vi "ReadTrajectory_JSON_File_WriteFGV_Example.vi"() -> ()   [LabVIEW 2019]
panel:
  out "error out":errorcluster
  # "Read Trajectory JSON File and Write to Functional Global Variable"
  # "See block diagram"
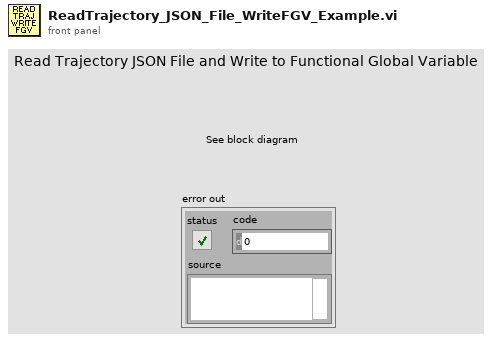
[diagram p1: front panel]
types:
  T1 = enum16{"Sample Fwd", "Sample Rev", "Read Traj", "Write Traj"}
  T2 = typedef "Trajectory_Library.lvlib/TRAJECTORY.ctl" = cluster{"TotalTImeSecs":dbl, "States":T3[]}
  T3 = typedef "Trajectory_Library.lvlib/TRAJ_STATE.ctl" = cluster{"TimeSeconds":dbl, "Velocity":dbl, "Acceleration":dbl, "POSE":T4, "Curvature":dbl}
  T4 = typedef "Trajectory_Library.lvlib/POSE2D.ctl" = cluster{"TRANSLATION":T5, "ROTATION":T6}
  T5 = typedef "Trajectory_Library.lvlib/TRANSLATION2D.ctl" = cluster{"X":dbl, "Y":dbl}
  T6 = typedef "Trajectory_Library.lvlib/ROTATION2D.ctl" = cluster{"VALUE":dbl, "COS":dbl, "SIN":dbl}
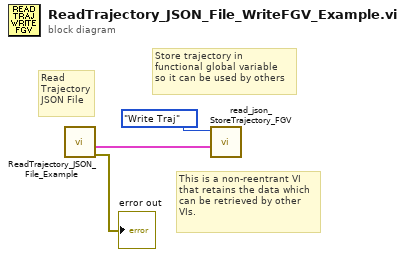
[diagram p0: block diagram]
diagram:
  # "This is a non-reentrant VI\nthat retains the data which\ncan be retrieved by other\nVIs."
  # "Read\nTrajectory\nJSON File"
  # "Store trajectory in\nfunctional global variable\nso it can be used by others"
  n1 = call "ReadTrajectory_JSON_File_Example.vi"() -> ("error out"=→"error out":errorcluster, "outTRAJECTORY"=w2:T2)  [unwired: 8 in, 2 out]
  n2 = call "read_json_StoreTrajectory_FGV.vi"("inTRAJECTORY"=w2, "Command"=T1."Write Traj") -> ()  [unwired: 8 in, 2 out]
